vi "Lecroy_fast_fetch_wfm.vi"(0 "VISA resource name":refnum<visa-resource-name>, 5 "Source (0: Channel 1)":u16(ring) items=["Channel 1", "Channel 2", "Channel 3", "Channel 4", "Memory 1", "Memory 2", "Memory 3", "Memory 4", "Function 1", "Function 2", "Function 3", "Function 4", "Function 5", "Function 6", "Function 7", "Function 8", "Other"], 8 "Custom Source ID":string, 9 "Timeout (10000 ms)":u32=10000, 11 "error in (no error)":errorcluster) -> (4 "VISA resource name out":refnum<visa-resource-name>, 6 "Waveform Graph":waveform(dbl)(graph), 10 "Number Of Data Points":u32, 15 "error out":errorcluster)   [LabVIEW 2013]
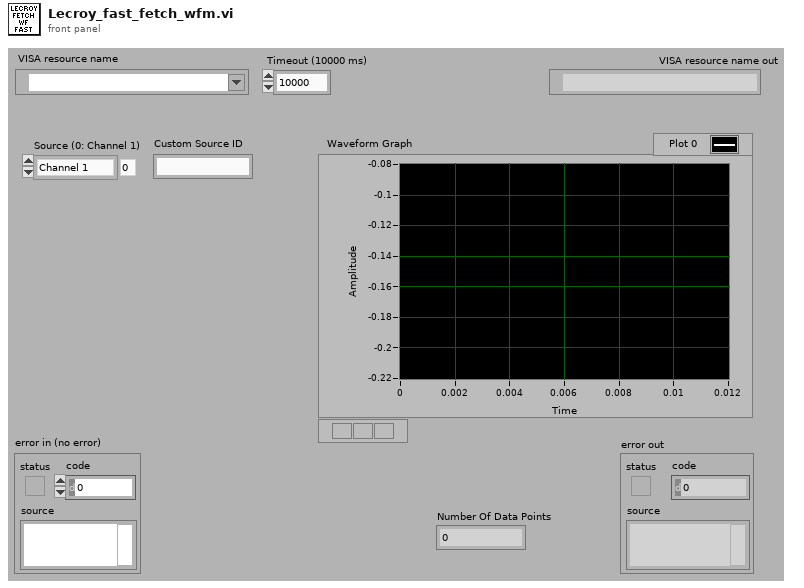
[diagram p1: front panel]
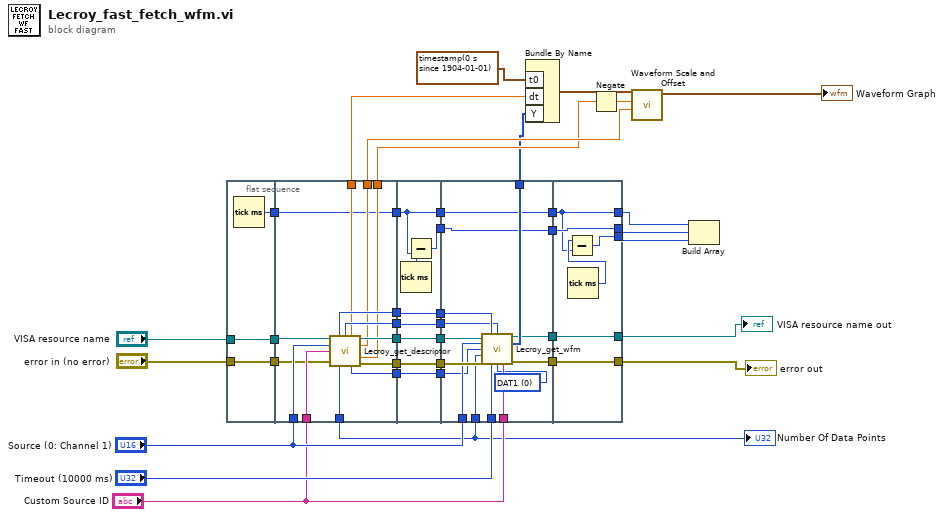
[diagram p0: block diagram]
diagram:
  n1 = flat-sequence {
    tunnel: [w42] -> w7
    tunnel: [w41] -> w5
    tunnel: "VISA resource name" -> [w41]
    tunnel: [w40] -> w3
    tunnel: "error in (no error)" -> [w40]
    tunnel: "Source (0: Channel 1)" -> [w56]
    tunnel: "Custom Source ID" -> [w55]
    tunnel: [w54] -> w35
    tunnel: [w53] -> w33
    tunnel: [w52] -> w30
    tunnel: [w51] -> w28
    tunnel: [w50] -> w25
    tunnel: [w49] -> w24
    tunnel: [w48] -> w23
    tunnel: [w47] -> w22
    tunnel: [w46] -> w8
    tunnel: w7 -> [w46]
    tunnel: w5 -> [w45]
    tunnel: w3 -> [w44]
    tunnel: [w43] -> w1
    tunnel: w35 -> [w64]
    tunnel: [w64] -> w34
    tunnel: w33 -> [w63]
    tunnel: [w63] -> w32
    tunnel: [w62] -> w31
    tunnel: w30 -> [w62]
    tunnel: [w61] -> w29
    tunnel: w28 -> [w61]
    tunnel: [w60] -> w26
    tunnel: w25 -> [w60]
    tunnel: [w58] -> w14
    tunnel: [w57] -> w9
    tunnel: w8 -> [w57]
    tunnel: w34 -> [w79]
    tunnel: w32 -> [w78]
    tunnel: w31 -> [w77]
    tunnel: w29 -> [w76]
    tunnel: "Source (0: Channel 1)" -> [w75]
    tunnel: w26 -> [w74]
    tunnel: w1 -> [w73]
    tunnel: [w72] -> w21
    tunnel: "Timeout (10000 ms)" -> [w71]
    tunnel: "Custom Source ID" -> [w70]
    tunnel: [w68] -> w18
    tunnel: [w67] -> w16
    tunnel: w14 -> [w66]
    tunnel: [w66] -> w13
    tunnel: [w65] -> w10
    tunnel: w9 -> [w65]
    tunnel: w18 -> [w85]
    tunnel: [w85] -> w17
    tunnel: w16 -> [w84]
    tunnel: [w84] -> w15
    tunnel: [w82] -> w12
    tunnel: w13 -> [w82]
    tunnel: [w81] -> w11
    tunnel: [w80] -> w6
    tunnel: w10 -> [w80]
    frame #0 {
      n2 = Tick Count (ms)() -> (millisecond timer value=w42:u32)
    }
    frame #1 {
      n3 = call "Lecroy_get_descriptor.vi"("VISA resource name"=w45, "Source (0: Channel 1)"=w56, "Custom Source ID"=w55, "error in (no error)"=w44) -> ("First Valid Point"=w54:u32, "Last Valid Point"=w53:u32, "Horizontal interval"=w49:sgl, "VISA resource name out"=w52:refnum<visa-resource-name>, "Vertical gain"=w48:sgl, "Vertical offset"=w47:sgl, "Number Of Data Points"=w43:u32, "Command type"=w50:u32, "error out"=w51:errorcluster)  [unwired: 3 out]
    }
    frame #2 {
      n4 = Tick Count (ms)() -> (millisecond timer value=w59:u32)
      n5 = Subtract(x=w59, y=w57) -> (x-y=w58:u32)
    }
    frame #3 {
      w69 = u32 0 items=["DAT1", "DAT2"] ("Array (1: DAT1)")
      n6 = call "Lecroy_get_wfm.vi"("VISA resource name"=w77, "First Valid Point"=w79, "Last Valid Point"=w78, "Source (0: Channel 1)"=w75, "Command type (0: byte)"=w74, "Number Of Data Points (10000)"=w73, "error in (no error)"=w76, "Timeout (10000 ms)"=w71, "Array (0: DAT1)"=w69, "Custom Source ID"=w70) -> ("VISA resource name out"=w68:refnum<visa-resource-name>, "Waveform Graph"=w72:i16[], "error out"=w67:errorcluster)  [unwired: 3 out]
    }
    frame #4 {
      n7 = Tick Count (ms)() -> (millisecond timer value=w83:u32)
      n8 = Subtract(x=w83, y=w80) -> (x-y=w81:u32)
    }
  }
  n9 = Bundle By Name ("Build Waveform")("t0"=timestamp(0 s since 1904-01-01), "dt"=w24, "Y"=w21) -> (w39:waveform(i16))  [unwired: 1 out]
  n10 = Negate(x=w22) -> (-x=w37:sgl)
  n11 = call <vilib>:"Waveform Scale and Offset.vi"("scale"=w23, "offset"=w37, "waveform in"=w39) -> ("waveform out"=→"Waveform Graph":waveform(dbl))  [unwired: 1 in, 7 out]
  n12 = Build Array(w6, w12, w11) -> ()  [unwired: 1 out]
  "VISA resource name out" <- w17
  "error out" <- w15
  "Number Of Data Points" <- w1
